vi "Prime BSI Camera Engine.vi"(0 "Notifier Name":string, 11 "Camera Index and Px Size":string[](array[string])) -> ()   [LabVIEW 2020]
uses:
  Prime BSI Type Defs/Prime BSI Parameters.ctl
  Prime BSI Type Defs/Prime BSI Parameter List.ctl
  Prime BSI Type Defs/Prime BSI ROI.ctl
  Prime BSI Type Defs/Prime BSI Notifier Element.ctl
  Prime BSI Type Defs/Prime BSI Actions.ctl
  <vilib>/vision/Image Controls.llb/IMAQ Image.ctl
  C:/Users/Public/Documents/Photometrics/TPM-LabVIEWSamples/Examples/2020/Dependencies/PVCamNET.dll
  Public/Documents/Photometrics/TPM-LabVIEWSamples/Examples/2020/Dependencies/PVCamNET.dll
  Camera Controls/Camera IMAQ Key Info.ctl
  shell32.dll
panel:
  out "Last Error":errorcluster
  out "Camera Name":string
  in  "Quit":bool
  in  "File Save Path":path
  in  "# of Frames":u32
  in  "Get ROI":bool
  in  "ROI Setup":T1
  in  "Set ROI":bool
  in  "PVCam Parameter":T2
  in  "Set Parameter":bool
  in  "Get Parameter":bool
  in  "Capture":bool
  in  "Live Preview":bool
  in  "Use Display Module":bool
  out "Frame":u32
  out "Image Key Error":errorcluster
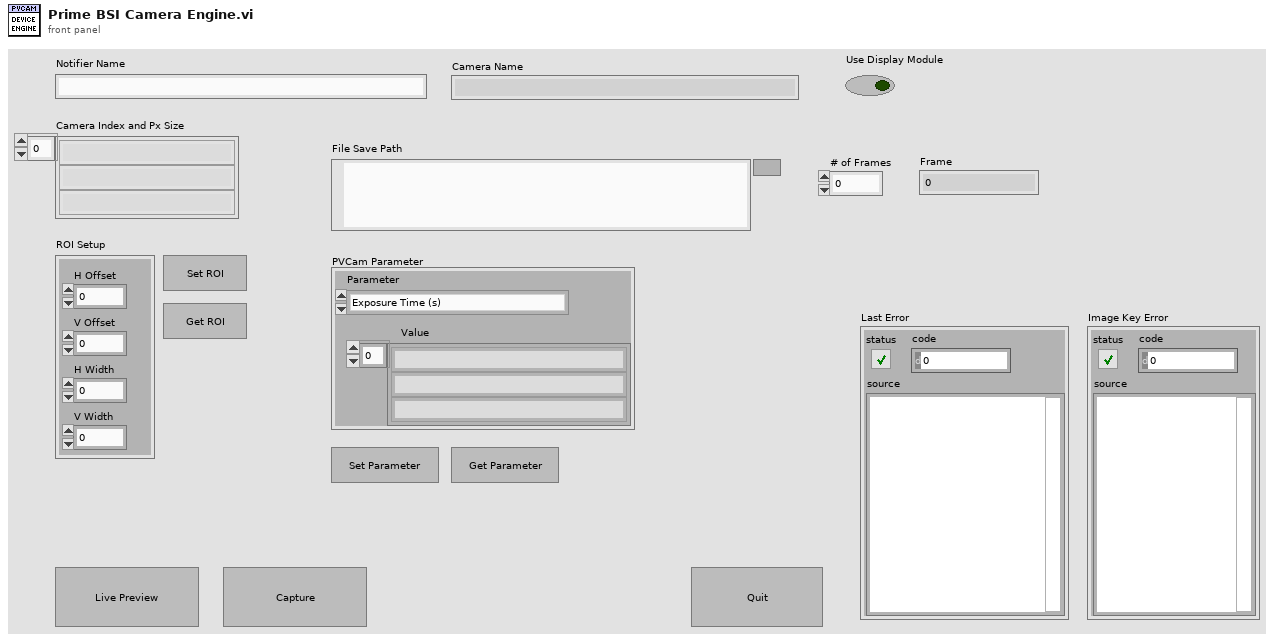
[diagram p1: front panel]
types:
  T1 = typedef "Prime BSI ROI.ctl" = cluster{"H Offset":i32, "V Offset":i32, "H Width":i32, "V Width":i32}
  T2 = typedef "Prime BSI Parameters.ctl" = cluster{"Parameter":T3, "Value":string[]}
  T3 = typedef "Prime BSI Parameter List.ctl" = enum16{"Exposure Time (s)", "Binning", "Readout Port List", "Available Gain List"}
  T4 = typedef "Image Type" = u32
  T5 = typedef "Prime BSI Actions.ctl" = enum16{"Do Nothing", "Preview", "Record", "Abort", "Record Settings", "Set Parameter", "Get Parameter", "Set ROI", "Get ROI", "Status", "Quit"}
  T6 = typedef "Prime BSI Notifier Element.ctl" = cluster{"PVCam Actions":T5, "Received?":bool, "PVCam Parameter":T2, "PVCam ROI":T1, "Running?":bool, "File Path":path, "# of frames":u32, "Image Ref":T7, "Binning":i32}
  T7 = typedef "IMAQ Image.ctl" = refnum<image>
  T8 = typedef "Camera IMAQ Key Info.ctl" = cluster{"Frame":u32, "Sensor Height":i32, "Sensor Width":i32, "ROI Height":i32, "ROI Width":i32, "ROI Enable?":bool, "Bit per Pixel":u8}
  T9 = enum32{"Invalid", "Standard", "Closed", "Hidden", "Minimized", "Maximized"}
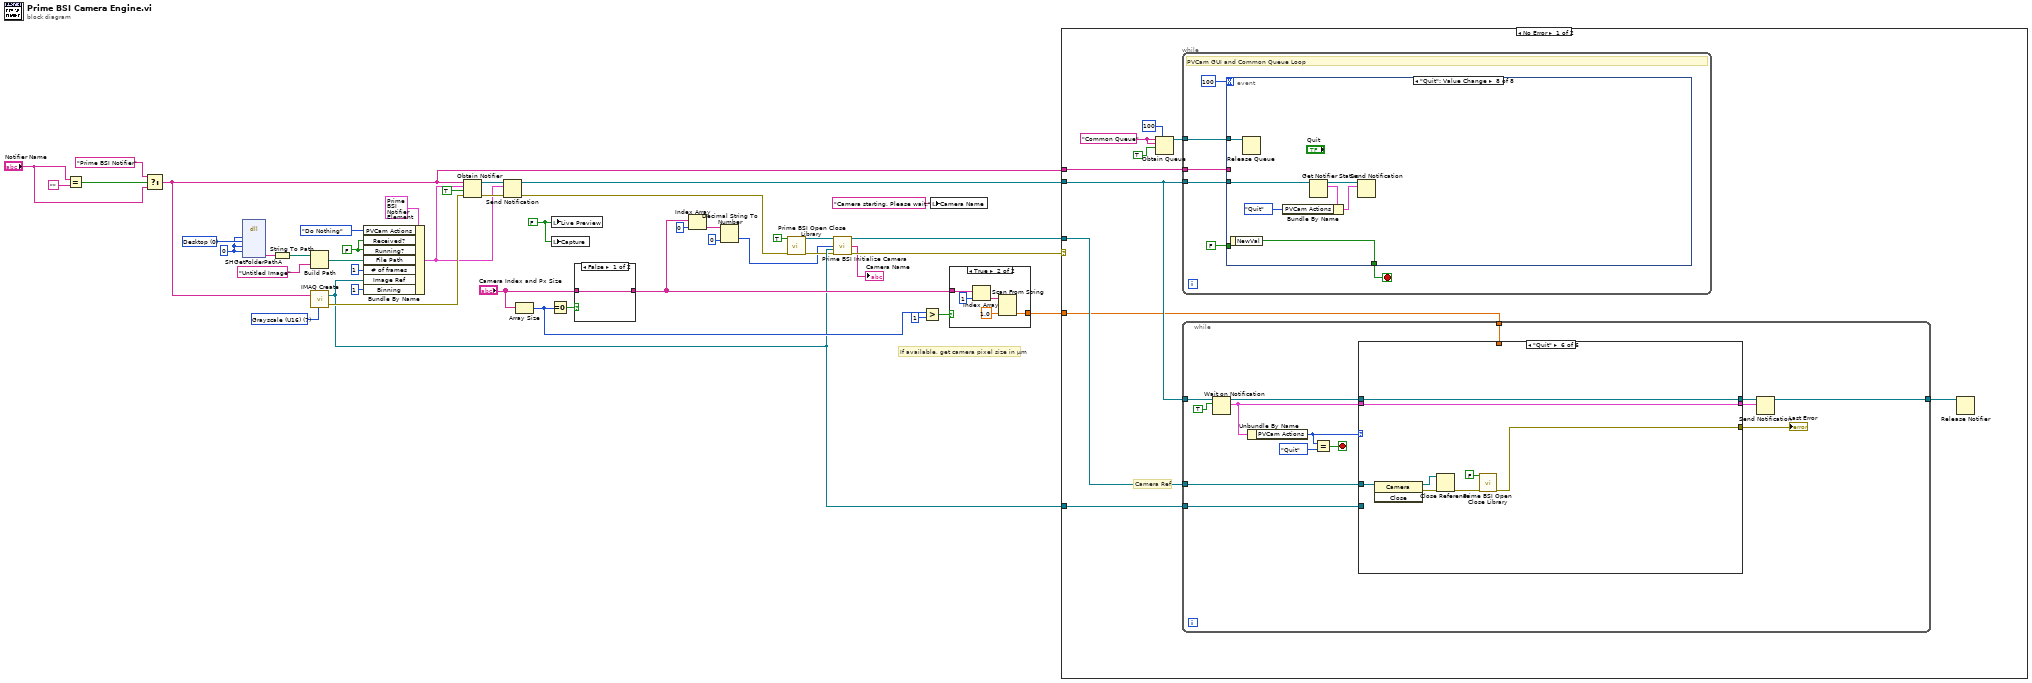
[diagram p0: block diagram]
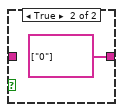
[diagram p2: hidden frame]
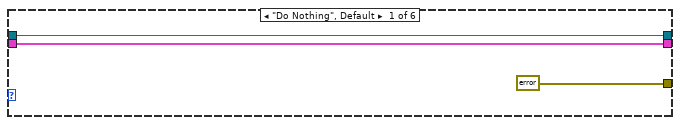
[diagram p3: hidden frame]
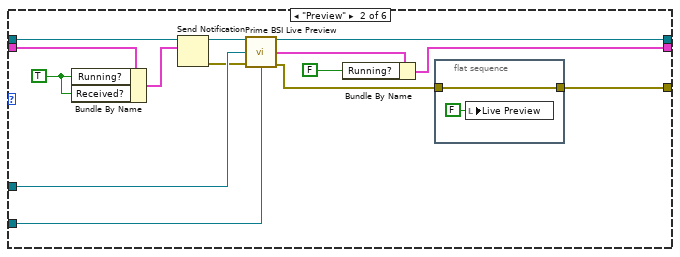
[diagram p4: hidden frame]
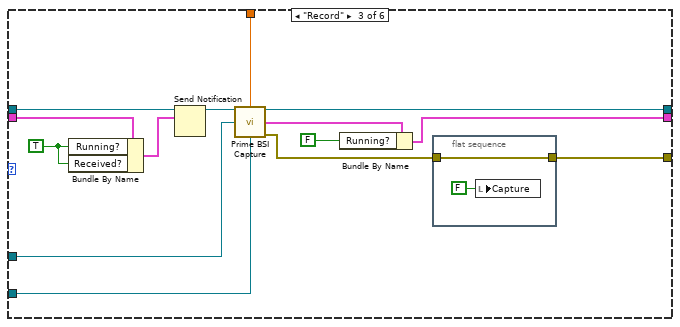
[diagram p5: hidden frame]
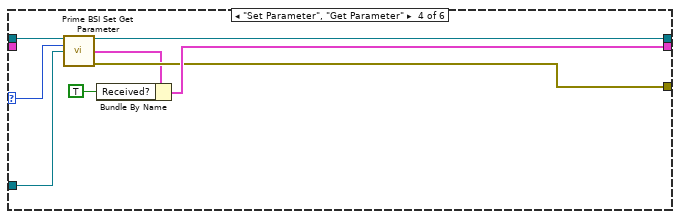
[diagram p6: hidden frame]
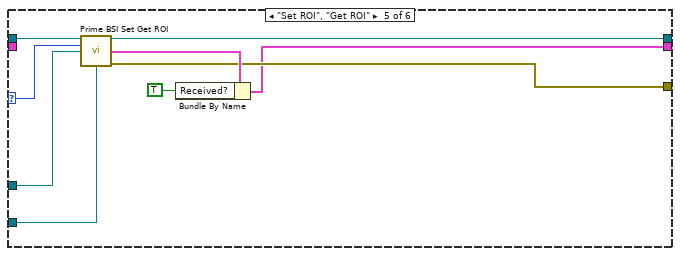
[diagram p7: hidden frame]
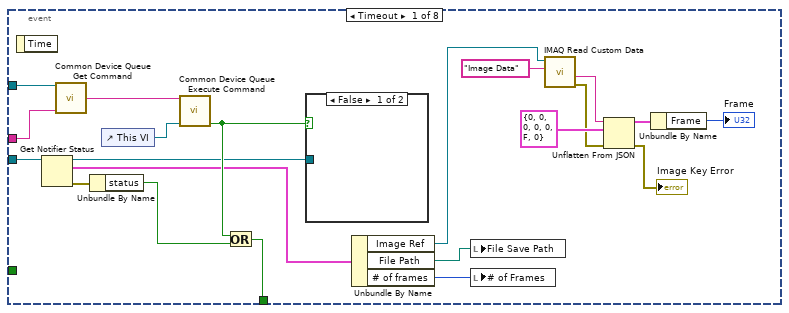
[diagram p8: hidden frame]
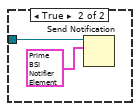
[diagram p9: hidden frame]
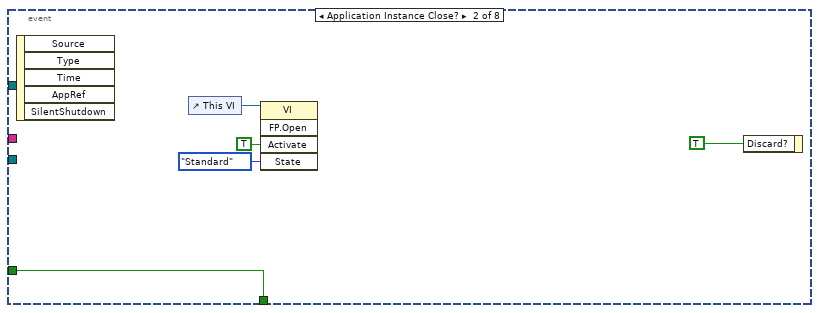
[diagram p10: hidden frame]
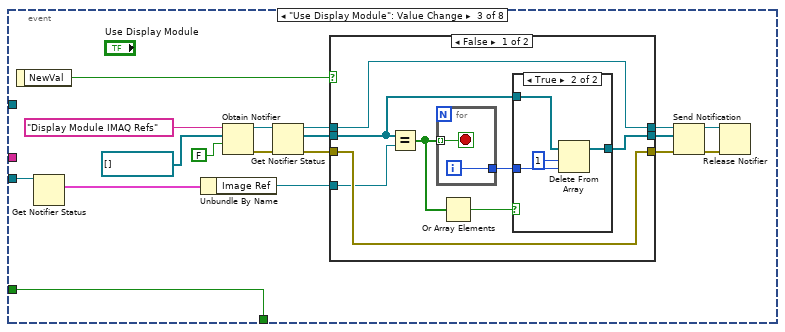
[diagram p11: hidden frame]
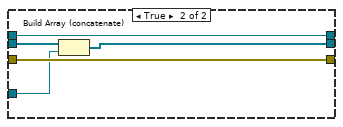
[diagram p13: hidden frame]
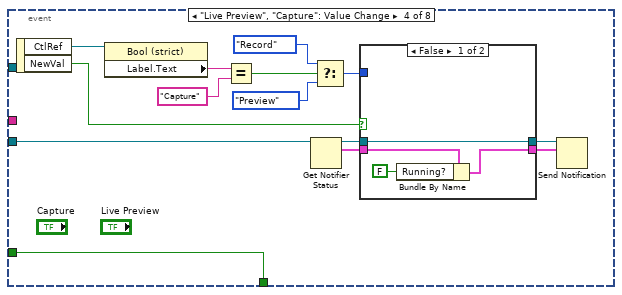
[diagram p14: hidden frame]
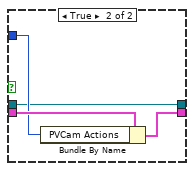
[diagram p15: hidden frame]
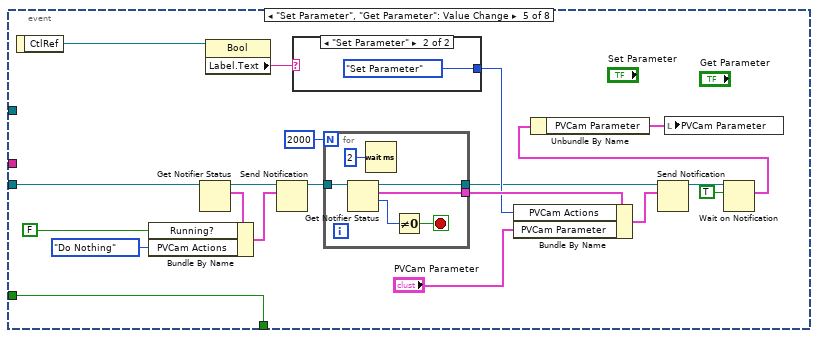
[diagram p16: hidden frame]
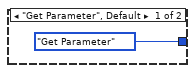
[diagram p17: hidden frame]
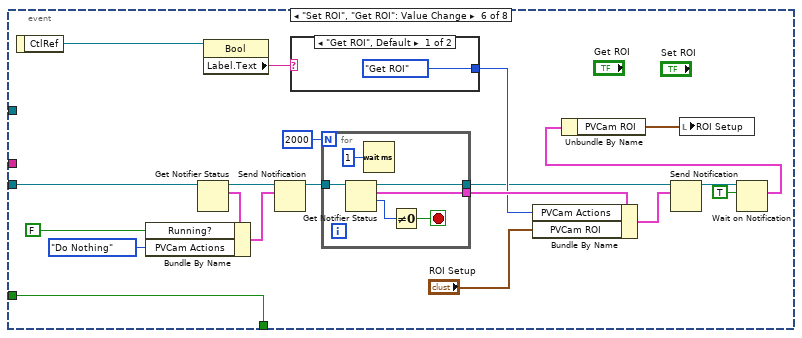
[diagram p18: hidden frame]
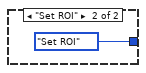
[diagram p19: hidden frame]
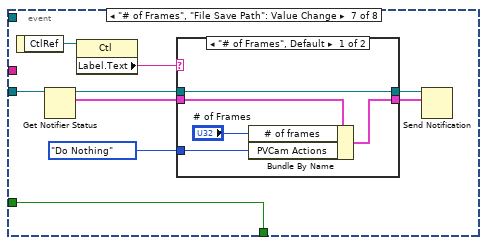
[diagram p20: hidden frame]
diagram:
  w9 = FALSE ("Live Preview")
  w28 = T4 7 items=["Grayscale (U8)", "Grayscale (I16)", "Grayscale (SGL)", "Complex (CSG)", "RGB (U32)", "HSL (U32)", "RGB (U64)", "Grayscale (U16)"] ("Image Type")
  w34 = 0 items=["Desktop"=0, "Personal Documents"=5, "AppData"=26, "Local AppData"=28, "Common AppData"=35, "Program Files"=38, "Program Files Common"=43, "Common Documents"=46] ("Requested Path")
  w33 = 0 ("HWND")
  w35 = FALSE ("Running?")
  # "If available, get camera pixel size in µm"
  n1 = Equal?(x="Notifier Name", y="") -> (x = y?=w17:bool)
  n2 = Select(t="Prime BSI Notifier", s=w17, f="Notifier Name") -> (s? t:f=w14:string)
  n3 = dll-call lib="shell32.dll" fn="SHGetFolderPathA"("HWND"=w33, "nFolder"=w34, "hToken"=w33, "dwFlags"=w33) -> ("pszPath"=w32:string)  [unwired: 9 in, 2 out]
  n4 = String To Path(string=w32) -> (path=w30:path)
  n5 = Build Path(base path=w30, name or relative path="Untitled Image") -> (appended path=w29:path)
  n6 = call "IMAQ Create"("Image Name"=w14, "Image Type"=w28) -> ("New Image"=w5:T7, "error out"=w27:errorcluster)  [unwired: 3 in]
  n7 = Bundle By Name(cluster=T6 {"PVCam Actions"=enum."Do Nothing", "Received?"=FALSE, "PVCam Parameter"={"Parameter"=enum."Exposure Time (s)", "Value"=[]}, "PVCam ROI"={"H Offset"=0, "V Offset"=0, "H Width"=0, "V Width"=0}, "Running?"=FALSE, "File Path"=path "", "# of frames"=0, "Image Ref"=refnum, "Binning"=0} ("IDS Camera Cluster"), "PVCam Actions"=Prime_BSI_Actions."Do Nothing", "Received?"=w35, "Running?"=w35, "File Path"=w29, "# of frames"=u32 1, "Image Ref"=w5, "Binning"=1) -> (w20:T6)
  n8 = Obtain Notifier(name (unnamed)=w14, notification data type=w20, create if not found? (T)=TRUE, error in (no error)=w27) -> (notifier out=w23:refnum<notifier>, error out=w22:errorcluster)  [unwired: 1 out]
  n9 = Send Notification(notification=w20, notifier=w23, error in (no error)=w22) -> (notifier out=w21:refnum<notifier>, error out=w4:errorcluster)
  n10 = Array Size(array="Camera Index and Px Size") -> (size(s)=w10:i32)
  n11 = Equal To 0?(x=w10) -> (x = 0?=w13:bool)
  n12 = local write "Live Preview"(w9) -> ()
  n13 = local write "Capture"(w9) -> ()
  n14 = case shown="False" w13 {
    tunnel: "Camera Index and Px Size" -> [w45 _]
    tunnel: [w45 string[] ["0"] ("Camera Index and Px Size")] -> w11
    frame False {
    }
    frame True {
    }
  }
  n15 = Index Array(array=w11, index=0) -> (element=w42:string)
  n16 = Decimal String To Number(string=w42, default (0L)=0 ("default (0 I32)")) -> (number=w2:i32)  [unwired: 1 in, 1 out]
  n17 = call "Prime BSI Open Close Library.vi"("Open Library?"=TRUE, "Error In"=w4) -> ("Cameras Ref"=w1:refnum<k24>, "Error Out"=w3:errorcluster)  [unwired: 11 in, 1 out]
  n18 = call "Prime BSI Initialize Camera.vi"("Cameras Ref"=w1, "Camera Index"=w2, "Image Ref"=w5, "Error In"=w3) -> ("Camera Ref"=w7:refnum<k24>, "Camera Name"=→"Camera Name":string, "Error Out"=w24:errorcluster)  [unwired: 9 in]
  n19 = Greater?(x=w10, y=1) -> (0:w41:bool)
  n20 = local write "Camera Name"("Camera starting. Please wait." ("Camera Name")) -> ()
  n21 = case shown="True" w41 {
    tunnel: w11 -> [_ w50]
    tunnel: [1.0 ("default (0 dbl)") w52] -> w25
    frame False {
    }
    frame True {
      n22 = Index Array(array=w50, index=1) -> (element=w51:string)
      n23 = Scan From String(input string=w51, default 1=1.0 ("default (0 dbl)")) -> (output 1=w52:dbl)  [unwired: 3 in, 3 out]
    }
  }
  n24 = case shown="No Error" w24 {
    selector: w24 -> [_ w317]
    tunnel: w21 -> [w57 w319]
    tunnel: w7 -> [w56 w318]
    tunnel: w25 -> [w53 _]
    tunnel: w14 -> [w58 _]
    tunnel: w5 -> [w55 _]
    frame No Error {
      w62 = "Common Queue" ("Unique Notifier Name")
      # "Camera Ref"
      n25 = Obtain Queue(max queue size (-1, unlimited)=100, name (unnamed)=w62, element data type=w62, create if not found? (T)=TRUE) -> (queue out=w59:refnum<queue>)  [unwired: 1 in, 2 out]
      n26 = while {
        tunnel: w59 -> [w141]
        tunnel: w58 -> [w139]
        tunnel: w57 -> [w140]
        stop <- w138 stop-if-true
        # "PVCam GUI and Common Queue Loop"
        n27 = event shown="[7] \"Quit\": Value Change" {
          selector: _ -> [_ _ _ _ _ _ _ _]
          dyn-events: _ -> [_ _ _ _ _ _ _ _]
          timeout: 100 -> [_ _ _ _ _ _ _ _]
          tunnel: w141 -> [w157 _ _ _ _ _ _ w312]
          tunnel: w140 -> [w156 _ w188 w215 w248 w276 w293 w311]
          tunnel: w139 -> [w155 _ _ _ _ _ _ _]
          tunnel: [w154 w170 w171 w222 w250 w278 w295 w307] -> w138
          tunnel: FALSE -> [_ w170 w171 w222 w250 w278 w295 _]
          event Timeout {
            n28 = event-data() -> ()  [unwired: 1 in, 1 out]
            n29 = Get Notifier Status(notifier=w156) -> (notifier out=w158:refnum<notifier>, current notification=w151:T6, error out=w163:errorcluster)  [unwired: 1 in, 2 out]
            n30 = call "Common Device Queue Get Command.vi"("Common Queue"=w157, "Notifier Name"=w155) -> ("Command"=w162:string)  [unwired: 12 in, 1 out]
            n31 = Unbundle By Name(w163) -> ("status"=w160:bool)
            n32 = control-ref of="This VI"() -> (w161:refnum<vi>)
            n33 = call "Common Device Queue Execute Command.vi"("Common Command"=w162, "VI Refnum"=w161) -> ("Quit?"=w159:bool)  [unwired: 12 in, 1 out]
            n34 = Or(x=w159, y=w160) -> (x .or. y?=w154:bool)
            n35 = case shown="False" w159 {
              tunnel: w158 -> [_ w165]
              frame False {
              }
              frame True {
                n36 = Send Notification(notification=T6 {"PVCam Actions"=enum."Quit", "Received?"=FALSE, "PVCam Parameter"={"Parameter"=enum."Exposure Time (s)", "Value"=[]}, "PVCam ROI"={"H Offset"=0, "V Offset"=0, "H Width"=0, "V Width"=0}, "Running?"=FALSE, "File Path"=path "", "# of frames"=0, "Image Ref"=refnum, "Binning"=0} ("IDS Camera Cluster"), notifier=w165) -> ()  [unwired: 1 in, 2 out]
              }
            }
            n37 = Unbundle By Name(w151) -> ("Image Ref"=w149:T7, "File Path"=w153:path, "# of frames"=w152:u32)
            n38 = local write "File Save Path"(w153) -> ()
            n39 = local write "# of Frames"(w152) -> ()
            n40 = call "IMAQ Read Custom Data"("Key"="Image Data", "Image"=w149) -> ("error out"=w144:errorcluster, "Custom Data Out"=w147:string)  [unwired: 7 in, 1 out]
            n41 = Unflatten From JSON(JSON string=w147, type and defaults=T8 {"Frame"=0, "Sensor Height"=0, "Sensor Width"=0, "ROI Height"=0, "ROI Width"=0, "ROI Enable?"=FALSE, "Bit per Pixel"=0} ("Camera IMAQ Key Info"), error in (no error)=w144) -> (value=w146:T8, error out=→"Image Key Error":errorcluster)  [unwired: 4 in]
            n42 = Unbundle By Name(w146) -> ("Frame"=→"Frame":u32)
          }
          event Application Instance Close? {
            n43 = event-data() -> ()  [unwired: 1 in, 5 out]
            n44 = control-ref of="This VI"() -> (w167:refnum<vi>)
            n45 = invoke class="VI" method="FP.Open"(reference=w167, "Activate"=TRUE ("Activate?"), "State"=T9."Standard") -> ()  [unwired: 2 in, 5 out]
            n46 = event-data("Discard?"=TRUE) -> ()  [unwired: 1 in, 1 out]
          }
          event "Use Display Module": Value Change {
            n47 = event-data() -> ("NewVal"=w173:bool)  [unwired: 1 in]
            n48 = Get Notifier Status(notifier=w188) -> (current notification=w187:T6)  [unwired: 1 in, 4 out]
            n49 = Unbundle By Name(w187) -> ("Image Ref"=w172:T7)
            n50 = Obtain Notifier(name (unnamed)="Display Module IMAQ Refs", notification data type=T7[] [], create if not found? (T)=FALSE) -> (notifier out=w180:refnum<notifier>, error out=w179:errorcluster)  [unwired: 1 in, 1 out]
            n51 = Get Notifier Status(notifier=w180, error in (no error)=w179) -> (notifier out=w181:refnum<notifier>, current notification=w183:T7[], error out=w182:errorcluster)  [unwired: 2 out]
            n52 = case shown="False" w173 {
              tunnel: w181 -> [w196 w206]
              tunnel: w182 -> [w190 w205]
              tunnel: w183 -> [w192 w208]
              tunnel: [w191 w207] -> w186
              tunnel: [w196 w206] -> w184
              tunnel: [w190 w205] -> w185
              tunnel: w172 -> [w189 w204]
              frame False {
                n53 = Equal?(x=w192, y=w189) -> (x = y?=w195:bool[])
                n54 = for {
                  tunnel: w195 -> [w203] mode=indexing
                  tunnel: [w202] -> w193
                  i -> [w202]
                  stop <- w203 stop-if-true
                }
                n55 = Or Array Elements(Boolean array=w195) -> (logical OR=w194:bool)
                n56 = case shown="True" w194 {
                  tunnel: w193 -> [_ w200]
                  tunnel: w192 -> [w197 w199]
                  tunnel: [w197 w198] -> w191
                  frame False {
                  }
                  frame True {
                    n57 = Delete From Array(array=w199, length=1, index=w200) -> (array with subset deleted=w198:T7[])  [unwired: 1 out]
                  }
                }
              }
              frame True {
                n58 = Build Array (concatenate)(w208, w204) -> (w207:T7[])
              }
            }
            n59 = Send Notification(notification=w186, notifier=w184, error in (no error)=w185) -> (notifier out=w178:refnum<notifier>, error out=w177:errorcluster)
            n60 = Release Notifier(notifier=w178, error in (no error)=w177) -> ()  [unwired: 1 in, 3 out]
          }
          event "Live Preview", "Capture": Value Change {
            n61 = event-data() -> ("CtlRef"=w221:refnum<vi>, "NewVal"=w217:bool)  [unwired: 1 in]
            n62 = property class="Bool (strict)"(reference=w221) -> ("Label.Text"=w220:string)  [unwired: 1 in, 2 out]
            n63 = Equal?(x=w220, y="Capture") -> (x = y?=w218:bool)
            n64 = Get Notifier Status(notifier=w215) -> (notifier out=w214:refnum<notifier>, current notification=w213:T6)  [unwired: 1 in, 3 out]
            n65 = Select(t=Prime_BSI_Actions."Record" ("PVCam Actions"), s=w218, f=Prime_BSI_Actions."Preview" ("PVCam Actions")) -> (s? t:f=w216:T5)
            n66 = case shown="False" w217 {
              tunnel: w216 -> [_ w229]
              tunnel: w214 -> [w224 w228]
              tunnel: w213 -> [w226 w230]
              tunnel: [w224 w228] -> w212
              tunnel: [w223 w227] -> w211
              frame False {
                n67 = Bundle By Name(cluster=w226, "Running?"=FALSE) -> (w223:T6)
              }
              frame True {
                n68 = Bundle By Name(cluster=w230, "PVCam Actions"=w229) -> (w227:T6)
              }
            }
            n69 = Send Notification(notification=w211, notifier=w212) -> ()  [unwired: 1 in, 2 out]
          }
          event "Set Parameter", "Get Parameter": Value Change {
            n70 = event-data() -> ("CtlRef"=w249:refnum<vi>)  [unwired: 1 in]
            n71 = Get Notifier Status(notifier=w248) -> (notifier out=w243:refnum<notifier>, current notification=w246:T6)  [unwired: 1 in, 3 out]
            n72 = Bundle By Name(cluster=w246, "Running?"=FALSE, "PVCam Actions"=Prime_BSI_Actions."Do Nothing") -> (w242:T6)
            n73 = property class="Bool"(reference=w249) -> ("Label.Text"=w247:string)  [unwired: 1 in, 2 out]
            n74 = Send Notification(notification=w242, notifier=w243) -> (notifier out=w241:refnum<notifier>)  [unwired: 1 in, 1 out]
            n75 = case shown="\"Set Parameter\"" w247 {
              tunnel: [Prime_BSI_Actions."Get Parameter" ("PVCam Actions") Prime_BSI_Actions."Set Parameter" ("PVCam Actions")] -> w238
              frame "Get Parameter", Default {
              }
              frame "Set Parameter" {
              }
            }
            n76 = for {
              N: 2000 -> [_]
              tunnel: w241 -> [w255]
              tunnel: [w254] -> w237
              tunnel: [w253] -> w240
              stop <- w251 stop-if-true
              n77 = Get Notifier Status(notifier=w255) -> (notifier out=w254:refnum<notifier>, current notification=w253:T6, # waiting=w252:i32)  [unwired: 1 in, 2 out]
              n78 = Wait (ms)(milliseconds to wait=u32 2) -> ()  [unwired: 1 out]
              n79 = Not Equal To 0?(x=w252) -> (x != 0?=w251:bool)
            }
            n80 = Bundle By Name(cluster=w240, "PVCam Actions"=w238, "PVCam Parameter"="PVCam Parameter") -> (w236:T6)
            n81 = Send Notification(notification=w236, notifier=w237) -> (notifier out=w235:refnum<notifier>)  [unwired: 1 in, 1 out]
            n82 = Wait on Notification(notifier=w235, ignore previous (F)=TRUE) -> (notification=w233:T6)  [unwired: 2 in, 3 out]
            n83 = Unbundle By Name(w233) -> ("PVCam Parameter"=w232:T2)
            n84 = local write "PVCam Parameter"(w232) -> ()
          }
          event "Set ROI", "Get ROI": Value Change {
            n85 = event-data() -> ("CtlRef"=w277:refnum<vi>)  [unwired: 1 in]
            n86 = Get Notifier Status(notifier=w276) -> (notifier out=w271:refnum<notifier>, current notification=w274:T6)  [unwired: 1 in, 3 out]
            n87 = Bundle By Name(cluster=w274, "Running?"=FALSE, "PVCam Actions"=Prime_BSI_Actions."Do Nothing") -> (w270:T6)
            n88 = property class="Bool"(reference=w277) -> ("Label.Text"=w275:string)  [unwired: 1 in, 2 out]
            n89 = Send Notification(notification=w270, notifier=w271) -> (notifier out=w269:refnum<notifier>)  [unwired: 1 in, 1 out]
            n90 = case shown="\"Get ROI\", Default" w275 {
              tunnel: [Prime_BSI_Actions."Get ROI" ("PVCam Actions") Prime_BSI_Actions."Set ROI" ("PVCam Actions")] -> w267
              frame "Get ROI", Default {
              }
              frame "Set ROI" {
              }
            }
            n91 = for {
              N: 2000 -> [_]
              tunnel: w269 -> [w283]
              tunnel: [w282] -> w266
              tunnel: [w281] -> w268
              stop <- w279 stop-if-true
              n92 = Get Notifier Status(notifier=w283) -> (notifier out=w282:refnum<notifier>, current notification=w281:T6, # waiting=w280:i32)  [unwired: 1 in, 2 out]
              n93 = Wait (ms)(milliseconds to wait=u32 1) -> ()  [unwired: 1 out]
              n94 = Not Equal To 0?(x=w280) -> (x != 0?=w279:bool)
            }
            n95 = Bundle By Name(cluster=w268, "PVCam Actions"=w267, "PVCam ROI"="ROI Setup") -> (w265:T6)
            n96 = Send Notification(notification=w265, notifier=w266) -> (notifier out=w264:refnum<notifier>)  [unwired: 1 in, 1 out]
            n97 = Wait on Notification(notifier=w264, ignore previous (F)=TRUE) -> (notification=w262:T6)  [unwired: 2 in, 3 out]
            n98 = Unbundle By Name(w262) -> ("PVCam ROI"=w261:T1)
            n99 = local write "ROI Setup"(w261) -> ()
          }
          event "# of Frames", "File Save Path": Value Change {
            n100 = event-data() -> ("CtlRef"=w294:refnum<vi>)  [unwired: 1 in]
            n101 = Get Notifier Status(notifier=w293) -> (notifier out=w291:refnum<notifier>, current notification=w290:T6)  [unwired: 1 in, 3 out]
            n102 = property class="Ctl"(reference=w294) -> ("Label.Text"=w292:string)  [unwired: 1 in, 2 out]
            n103 = case shown="\"# of Frames\", Default" w292 {
              tunnel: w291 -> [w298 w305]
              tunnel: w290 -> [w300 w304]
              tunnel: [w298 w305] -> w289
              tunnel: [w297 w303] -> w288
              tunnel: Prime_BSI_Actions."Do Nothing" ("PVCam Actions") -> [w296 w301]
              frame "# of Frames", Default {
                n104 = Bundle By Name(cluster=w300, "# of frames"="# of Frames", "PVCam Actions"=w296) -> (w297:T6)
              }
              frame "File Save Path" {
                n105 = Bundle By Name(cluster=w304, "File Path"="File Save Path", "PVCam Actions"=w301) -> (w303:T6)
              }
            }
            n106 = Send Notification(notification=w288, notifier=w289) -> ()  [unwired: 1 in, 2 out]
          }
          event "Quit": Value Change {
            n107 = event-data() -> ("NewVal"=w307:bool)  [unwired: 1 in]
            n108 = Release Queue(queue=w312) -> ()  [unwired: 2 in, 3 out]
            n109 = Get Notifier Status(notifier=w311) -> (notifier out=w310:refnum<notifier>, current notification=w309:T6)  [unwired: 1 in, 3 out]
            n110 = Bundle By Name(cluster=w309, "PVCam Actions"=Prime_BSI_Actions."Quit") -> (w308:T6)
            n111 = Send Notification(notification=w308, notifier=w310) -> ()  [unwired: 1 in, 2 out]
          }
        }
      }
      n112 = while {
        tunnel: w57 -> [w75]
        tunnel: w56 -> [w69]
        tunnel: w55 -> [w68]
        tunnel: [w65] -> w54
        tunnel: w53 -> [w63]
        stop <- w73 stop-if-true
        n113 = Wait on Notification(notifier=w75, ignore previous (F)=TRUE) -> (notifier out=w71:refnum<notifier>, notification=w70:T6)  [unwired: 2 in, 2 out]
        n114 = Unbundle By Name(w70) -> ("PVCam Actions"=w72:T5)
        n115 = Equal?(x=w72, y=Prime_BSI_Actions."Quit") -> (x = y?=w73:bool)
        n116 = case shown="\"Quit\"" w72 {
          selector: w72 -> [_ _ _ w117 w122 _]
          tunnel: w71 -> [w79 w91 w108 w119 w127 w135]
          tunnel: w70 -> [w78 w89 w106 _ _ w134]
          tunnel: w69 -> [_ w93 w103 w118 w121 w136]
          tunnel: w68 -> [_ w85 w104 _ w120 _]
          tunnel: [w79 w92 w102 w114 w126 w135] -> w67
          tunnel: [w78 w83 w100 w115 w123 w134] -> w66
          tunnel: [errorcluster {"status"=FALSE, "code"=0, "source"=""} ("error out") w81 w97 w113 w124 w132] -> w64
          tunnel: w63 -> [_ _ w96 _ _ _]
          frame "Do Nothing", Default {
          }
          frame "Preview" {
            w88 = TRUE ("Running?")
            n117 = Bundle By Name(cluster=w89, "Running?"=w88, "Received?"=w88) -> (w87:T6)
            n118 = Send Notification(notification=w87, notifier=w91) -> (notifier out=w90:refnum<notifier>, error out=w86:errorcluster)  [unwired: 1 in]
            n119 = call "Prime BSI Live Preview.vi"("Notifier In"=w90, "Camera Ref"=w93, "Error In"=w86, "Image Ref"=w85) -> ("Notifier Out"=w92:refnum<notifier>, "Prime Cluster"=w84:T6, "Error Out"=w80:errorcluster)  [unwired: 9 in]
            n120 = Bundle By Name(cluster=w84, "Running?"=FALSE) -> (w83:T6)
            n121 = flat-sequence {
              tunnel: [w95] -> w81
              tunnel: w80 -> [w95]
              frame #0 {
                n122 = local write "Live Preview"(FALSE ("Live Preview")) -> ()
              }
            }
          }
          frame "Record" {
            w109 = TRUE ("Running?")
            n123 = Bundle By Name(cluster=w106, "Running?"=w109, "Received?"=w109) -> (w105:T6)
            n124 = Send Notification(notification=w105, notifier=w108) -> (notifier out=w107:refnum<notifier>)  [unwired: 1 in, 1 out]
            n125 = call "Prime BSI Capture.vi"("Notifier In"=w107, "Pixel Size"=w96, "Camera Ref"=w103, "Image Ref"=w104) -> ("Notifier Out"=w102:refnum<notifier>, "Prime Cluster"=w101:T6, "Error Out"=w98:errorcluster)  [unwired: 9 in]
            n126 = Bundle By Name(cluster=w101, "Running?"=FALSE) -> (w100:T6)
            n127 = flat-sequence {
              tunnel: w98 -> [w111]
              tunnel: [w111] -> w97
              frame #0 {
                n128 = local write "Capture"(FALSE ("Capture")) -> ()
              }
            }
          }
          frame "Set Parameter", "Get Parameter" {
            n129 = call "Prime BSI Set Get Parameter.vi"("Notifier In"=w119, "PVCam Actions"=w117, "Camera Ref"=w118) -> ("Notifier Out"=w114:refnum<notifier>, "PVCam Cluster"=w112:T6, "Error Out"=w113:errorcluster)  [unwired: 10 in]
            n130 = Bundle By Name(cluster=w112, "Received?"=TRUE) -> (w115:T6)
          }
          frame "Set ROI", "Get ROI" {
            n131 = call "Prime BSI Set Get ROI.vi"("Notifier In"=w127, "PVCam Actions"=w122, "Camera Ref"=w121, "Image Ref"=w120) -> ("Notifier Out"=w126:refnum<notifier>, "PVCam Cluster"=w125:T6, "Error Out"=w124:errorcluster)  [unwired: 9 in]
            n132 = Bundle By Name(cluster=w125, "Received?"=TRUE) -> (w123:T6)
          }
          frame "Quit" {
            n133 = invoke class="Camera" method="Close"(reference=w136) -> (reference out=w131:refnum<k24>, error out=w130:errorcluster)  [unwired: 2 in, 1 out]
            n134 = Close Reference(reference=w131, error in (no error)=w130) -> (error out=w129:errorcluster)
            n135 = call "Prime BSI Open Close Library.vi"("Open Library?"=FALSE, "Error In"=w129) -> ("Error Out"=w132:errorcluster)  [unwired: 11 in, 2 out]
          }
        }
        "Last Error" <- w64
        n136 = Send Notification(notification=w66, notifier=w67) -> (notifier out=w65:refnum<notifier>)  [unwired: 1 in, 1 out]
      }
      n137 = Release Notifier(notifier=w54) -> ()  [unwired: 2 in, 3 out]
    }
    frame Error {
      n138 = invoke class="Camera" method="Close"(reference=w318, error in=w317) -> (error out=w314:errorcluster)  [unwired: 1 in, 2 out]
      n139 = One Button Dialog(message="PVCam startup error.") -> ()  [unwired: 1 in, 1 out]
      n140 = call "Prime BSI Open Close Library.vi"("Open Library?"=FALSE, "Error In"=w314) -> ("Error Out"=w313:errorcluster)  [unwired: 11 in, 2 out]
      n141 = Release Notifier(notifier=w319, error in (no error)=w313) -> (error out=w316:errorcluster)  [unwired: 1 in, 2 out]
      n142 = local write "Last Error"(w316) -> ()
    }
  }
